vi "RichToFlatcif_common_Version.vi"(5 "OutputClusterType":T1, 11 "InputCluster":T2) -> (3 "OutputCluster":T1)   [LabVIEW 2021, in "Template_client.lvlib"]
uses:
  Template_client.lvlib
  cif_common_Version.ctl
  cif_common_Version_Flat.ctl
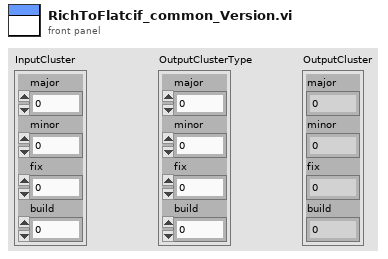
[diagram p1: front panel]
types:
  T1 = typedef "Template_client.lvlib/cif_common_Version_Flat.ctl" = cluster{"major":u32, "minor":u32, "fix":u32, "build":u32}
  T2 = typedef "Template_client.lvlib/cif_common_Version.ctl" = cluster{"major":u32, "minor":u32, "fix":u32, "build":u32}
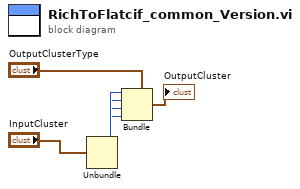
[diagram p0: block diagram]
diagram:
  n1 = Unbundle "Unbundle"("InputCluster") -> ("major"=w4:u32, "minor"=w3:u32, "fix"=w2:u32, "build"=w1:u32)
  n2 = Bundle "Bundle"(cluster="OutputClusterType", "major"=w4, "minor"=w3, "fix"=w2, "build"=w1) -> (→"OutputCluster":T1)
